vi "wait_for_hts_pump.vi"(8 "error in (no error)":errorcluster, 10 "PUMP":enum16{"PUMP2", "PUMP1"}(ring), 11 "HTS PORT IN":refnum<visa-resource-name>) -> (0 "error out":errorcluster, 3 "HTS PORT OUT":refnum<visa-resource-name>)   [LabVIEW 2013]
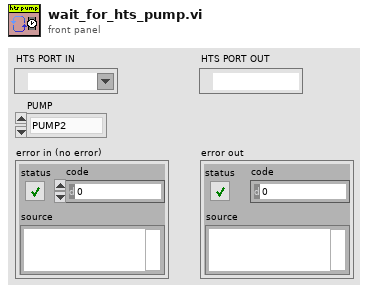
[diagram p1: front panel]
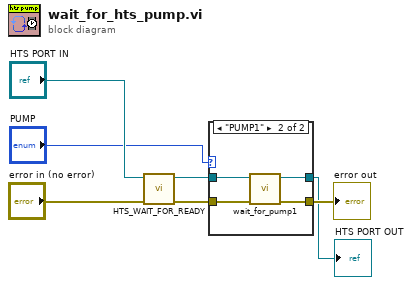
[diagram p0: block diagram]
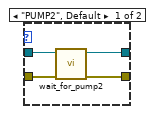
[diagram p2: hidden frame]
diagram:
  n1 = call "HTS_WAIT_FOR_READY.vi"("Error IN"="error in (no error)", "VISA resource IN"="HTS PORT IN") -> ("Error OUT"=w6:errorcluster, "VISA resource OUT"=w3:refnum<visa-resource-name>)  [unwired: 6 in, 2 out]
  n2 = case shown="\"PUMP1\"" "PUMP" {
    tunnel: [w8 w15] -> w7
    tunnel: w6 -> [w9 w14]
    tunnel: [w10 w13] -> w4
    tunnel: w3 -> [w11 w12]
    frame "PUMP2", Default {
      n3 = call "wait_for_pump2.vi"("error in (no error)"=w9, "HTS PORT IN"=w11) -> ("error out"=w8:errorcluster, "HTS PORT OUT"=w10:refnum<visa-resource-name>)  [unwired: 8 in]
    }
    frame "PUMP1" {
      n4 = call "wait_for_pump1.vi"("error in (no error)"=w14, "HTS PORT IN"=w12) -> ("error out"=w15:errorcluster, "HTS PORT OUT"=w13:refnum<visa-resource-name>)  [unwired: 8 in]
    }
  }
  "error out" <- w7
  "HTS PORT OUT" <- w4
